vi "Test 5 Get Type Full House with Joker.vi"(8 "error in (no error)":errorcluster, 11 "Test Case In":refnum<class "Day 7 Test.lvclass">) -> (0 "error out":errorcluster, 3 "Test Case Out":refnum<class "Day 7 Test.lvclass">)   [LabVIEW 2020, in "Day 7 Test.lvclass"]
uses:
  Day 7 Test.lvclass
  C:/Program Files (x86)/National Instruments/LabVIEW 2020/vi.lib/Astemes/LUnit/Test Case.lvclass
  <vilib>/Astemes/LUnit/Test Case.lvclass/Test Case.ctl
  ffb4b03f-324e-4da4-84c3-4c0cc3f10137.vi
  <vilib>/Astemes/LUnit/Append Pass Result.vi
  <vilib>/Astemes/LUnit/Append Fail Result.vi
  <vilib>/Astemes/LUnit/Describe Comparison.vi
  <vilib>/Astemes/LUnit/Compare Variants.vi
  <vilib>/Astemes/LUnit/Variant to string.vi
  <vilib>/Utility/Data Type/Get Type Information.vi
  <vilib>/Utility/LVClass/Get LV Class Name.vi
  Hand with Joker/Hand with Joker.lvclass
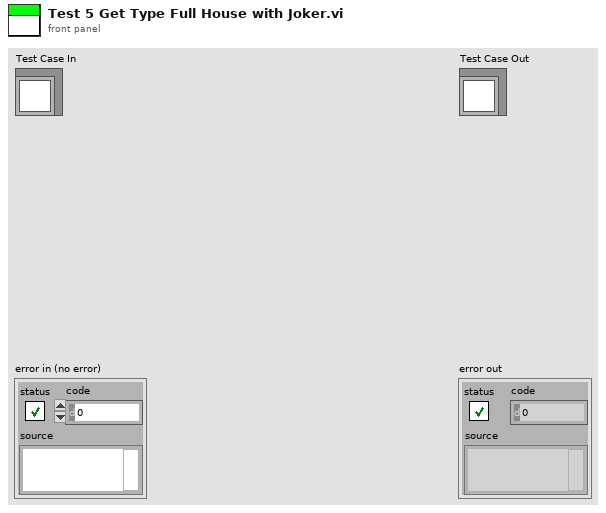
[diagram p1: front panel]
types:
  T1 = enum16{"High Card", "One Pair", "Two Pairs", "Three of a Kind", "Full House", "Four of a Kind", "Five of a Kind"}
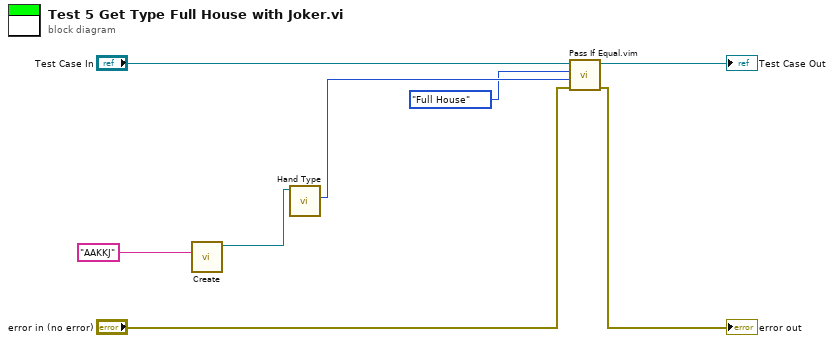
[diagram p0: block diagram]
diagram:
  n1 = call "Create.vi"("Input"="AAKKJ") -> ("Hand"=w3:refnum<class "Hand with Joker.lvclass">)  [unwired: 9 in, 1 out]
  n2 = call "Hand Type.vi"("Hand In"=w3) -> ("Score"=w2:T1)  [unwired: 8 in, 2 out]
  n3 = call "Pass If Equal.vim"("error in (no error)"="error in (no error)", "Actual"=w2, "Expected"=T1."Full House" ("Score"), "LUnit Test Case In"="Test Case In") -> ("error out"=→"error out":errorcluster, "LUnit Test Case Out"=→"Test Case Out":refnum<class "Day 7 Test.lvclass">)  [unwired: 6 in]
